vi "Load App.vi"   [LabVIEW 2021, in "OPC Server.lvlib" / "OPC Server.lvclass"]
doc: "Load the application into memory and start it running. The input notifier is used to send text to the splash screen to tell the user what stage the load process is in."
uses:
  OPC Server.lvclass
  C:/Program Files/National Instruments/LabVIEW 2021/vi.lib/ActorFramework/Actor/Actor.lvclass
  <vilib>/ActorFramework/Actor/Actor.lvclass
panel:
  # "OPC UA \nSimServer"
  # "Jung Lee"
types:
  T1 = enum32{"Invalid", "Standard", "Closed", "Hidden", "Minimized", "Maximized"}
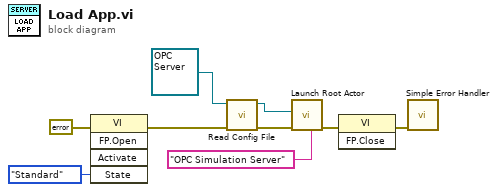
[diagram p0: block diagram]
diagram:
  n1 = invoke class="VI" method="FP.Open"(error in=errorcluster {"status"=FALSE, "code"=0, "source"=""} ("error in (no error)"), "State"=T1."Standard") -> (error out=w6:errorcluster)  [unwired: 3 in, 4 out]
  n2 = call "Read Config File.vi"("error in (no error)"=w6, "SM EOL Station Actor in"=refnum<class "OPC Server.lvclass"> refnum ("SM EOL Station Actor.lvlib:SM EOL Station Actor.lvclass")) -> ("error out"=w8:errorcluster, "SM EOL Station Actor out"=w7:refnum<class "OPC Server.lvclass">)  [unwired: 8 in]
  n3 = call <vilib>:"Launch Root Actor.vi"("Debug Alias"="OPC Simulation Server", "error in (no error)"=w8, "Actor"=w7) -> ("error out"=w2:errorcluster)  [unwired: 7 in, 1 out]
  n4 = invoke class="VI" method="FP.Close"(error in=w2) -> (error out=w1:errorcluster)  [unwired: 2 in, 2 out]
  n5 = call <vilib>:"Simple Error Handler.vi"("error in (no error)"=w1) -> ()  [unwired: 4 in, 5 out]
